vi "Read_Excel.vi"(11 "路径":path) -> (3 "表格控件":string[][](table))   [LabVIEW 2020]
panel:
  in  "Excel._Worksheet":refnum<k7>
  in  "Excel._Application":refnum<k7>
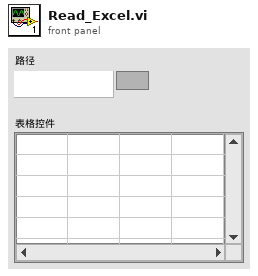
[diagram p1: front panel]
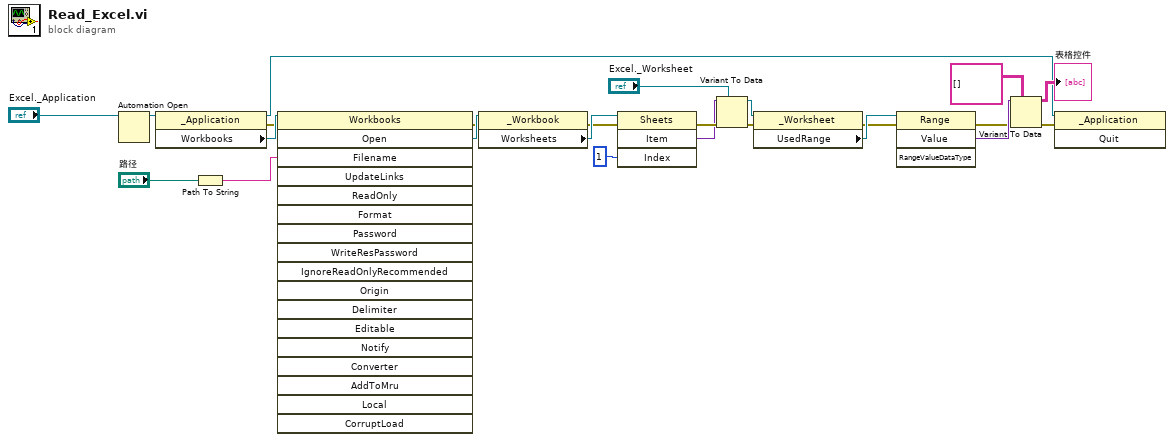
[diagram p0: block diagram]
diagram:
  n1 = Automation Open(Automation Refnum="Excel._Application") -> (Automation Refnum=w24:refnum<k7>)  [unwired: 3 in, 1 out]
  n2 = property class="_Application"(reference=w24) -> (reference out=w4:refnum<k7>, error out=w22:errorcluster, "Workbooks"=w23:refnum<k7>)  [unwired: 1 in]
  n3 = Path To String(path="路径") -> (string=w20:string)
  n4 = invoke class="Workbooks" method="Open"(reference=w23, error in=w22, "Filename"=w20) -> (error out=w18:errorcluster, "Open"=w19:refnum<k7>)  [unwired: 15 in, 16 out]
  n5 = property class="_Workbook"(reference=w19, error in=w18) -> (error out=w15:errorcluster, "Worksheets"=w16:refnum<k7>)  [unwired: 1 out]
  n6 = invoke class="Sheets" method="Item"(reference=w16, error in=w15, "Index"=1) -> (error out=w6:errorcluster, "Item"=w5:variant)  [unwired: 1 in, 2 out]
  n7 = Variant To Data(error in=w6, type="Excel._Worksheet", Variant=w5) -> (data=w2:refnum<k7>, error out=w14:errorcluster)
  n8 = property class="_Worksheet"(reference=w2, error in=w14) -> (error out=w12:errorcluster, "UsedRange"=w13:refnum<k7>)  [unwired: 1 out]
  n9 = invoke class="Range" method="Value"(reference=w13, error in=w12) -> (error out=w1:errorcluster, "Value"=w11:variant)  [unwired: 2 in, 2 out]
  n10 = Variant To Data(error in=w1, type=string[][] [], Variant=w11) -> (data=→"表格控件":string[][], error out=w7:errorcluster)
  n11 = invoke class="_Application" method="Quit"(reference=w4, error in=w7) -> ()  [unwired: 1 in, 3 out]
